vi "Write Session Handle.vi"(8 "error in (no error)":errorcluster, 10 "Session Handle":T1, 11 "Nephelometer in":refnum<class "Nephelometer.lvclass">) -> (0 "error out":errorcluster, 3 "Nephelometer out":refnum<class "Nephelometer.lvclass">)   [LabVIEW 2014, in "Nephelometer.lvclass"]
uses:
  Nephelometer.lvclass
  <userlib>/_Session Fwk/Typedefs/Session Handle.ctl
  <userlib>/_Session Fwk/Session - Root.lvclass
  Nephelometer.lvclass/Nephelometer.ctl
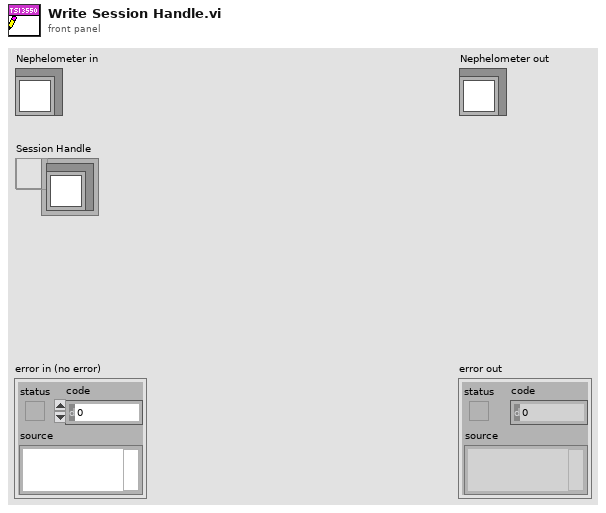
[diagram p1: front panel]
types:
  T1 = typedef "Session - Root.lvclass/Session Handle.ctl" = refnum<data-value>
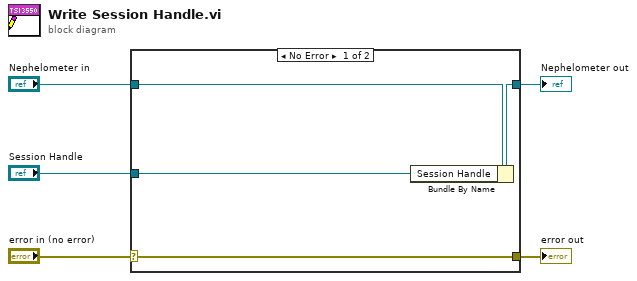
[diagram p0: block diagram]
diagram:
  n1 = case shown="No Error" "error in (no error)" {
    selector: "error in (no error)" -> [w9 w10]
    tunnel: [w9 w10] -> w4
    tunnel: [w7 w11] -> w2
    tunnel: "Nephelometer in" -> [w8 w11]
    tunnel: "Session Handle" -> [w6 _]
    frame No Error {
      n2 = Bundle By Name(cluster=w8, "Session Handle"=w6) -> (w7:refnum<class "Nephelometer.lvclass">)
    }
    frame Error {
    }
  }
  "error out" <- w4
  "Nephelometer out" <- w2
